vi "国弘探头清洗间隔.vi"(7 "探头":T1(ring)=enum."ORP", 8 "error in (no error)":errorcluster caption="错误输入（无错误）", 11 "清洗间隔":u16) -> (0 "error out":errorcluster caption="错误输出", 3 "MB session out":refnum<class "MB_Master.lvclass">)   [LabVIEW 2016, in "斯坦道多参数.lvlib"]
uses:
  <vilib>/Plasmionique/MB Master/MB_Master/MB_Master.lvclass
  <vilib>/Plasmionique/MB Master/MB Master.lvlib
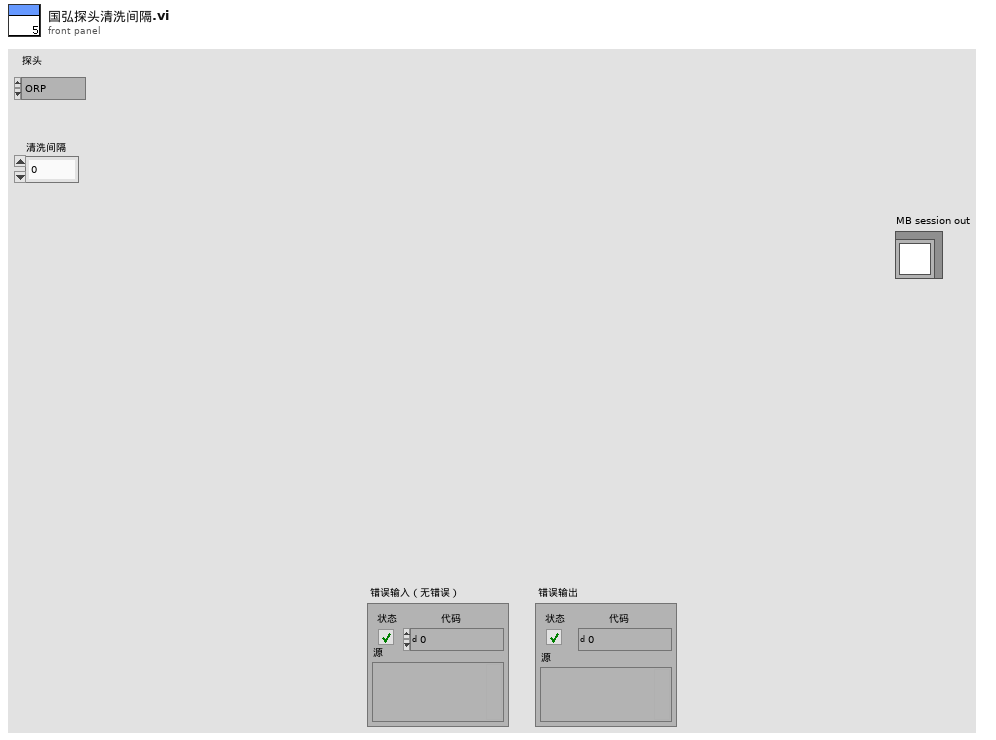
[diagram p1: front panel]
types:
  T1 = enum16{"NULL", "pH", "Cond", "DO", "Turb", "ORP"}
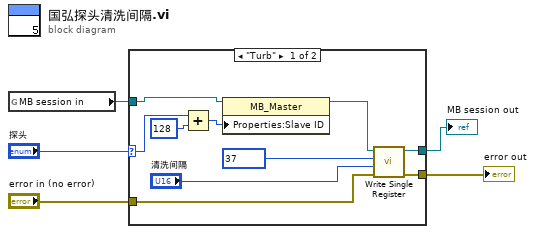
[diagram p0: block diagram]
diagram:
  n1 = global read "多参数全局变量.vi" "MB session in"() -> (w1:refnum<class "MB_Master.lvclass">)
  n2 = case shown="\"Turb\"" "探头" {
    selector: "探头" -> [w7 _]
    tunnel: "error in (no error)" -> [w14 w16]
    tunnel: w1 -> [w10 w17]
    tunnel: [w9 w16] -> w4
    tunnel: [w8 w17] -> w3
    frame "Turb" {
      n3 = Add(x=w7, y=u16 128) -> (x+y=w13:u16)
      n4 = property class="MB_Master"(reference=w10, "Properties:Slave ID"=w13) -> (reference out=w11:refnum<class "MB_Master.lvclass">)  [unwired: 1 in, 1 out]
      n5 = call <vilib>:"Write Single Register.vi"("error in (no error)"=w14, "value"="清洗间隔", "address"=u16 37 ("starting address"), "MB session in"=w11) -> ("error out"=w9:errorcluster, "MB session out"=w8:refnum<class "MB_Master.lvclass">)  [unwired: 6 in]
    }
    frame "NULL", Default {
    }
  }
  "error out" <- w4
  "MB session out" <- w3
